vi "SetWindowIcon.vi"(7 "Action":enum16{"Set", "Reset"}(ring), 8 "error in (no error)":errorcluster, 10 "VIRef (calling VI)":refnum<vi>, 11 "ICO Icon":path) -> (0 "Error Out":errorcluster)   [LabVIEW 2022 SP3]
doc: "Set a custom title bar icon for the referenced VI.\nIf no VI reference is supplied the VI calling this function is altered.\n\nUse <b>set</b> to change the icon to a custom icon, and <b>reset</b> to revert the icon to the previous value."
uses:
  user32.dll
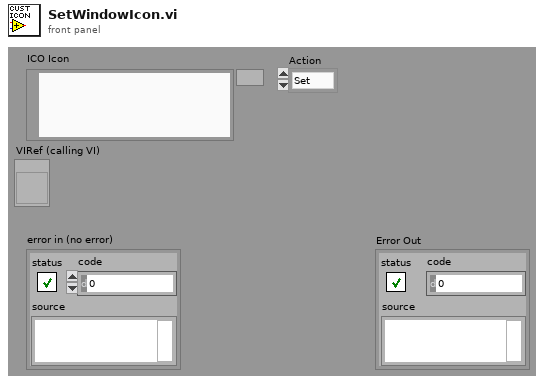
[diagram p1: front panel]
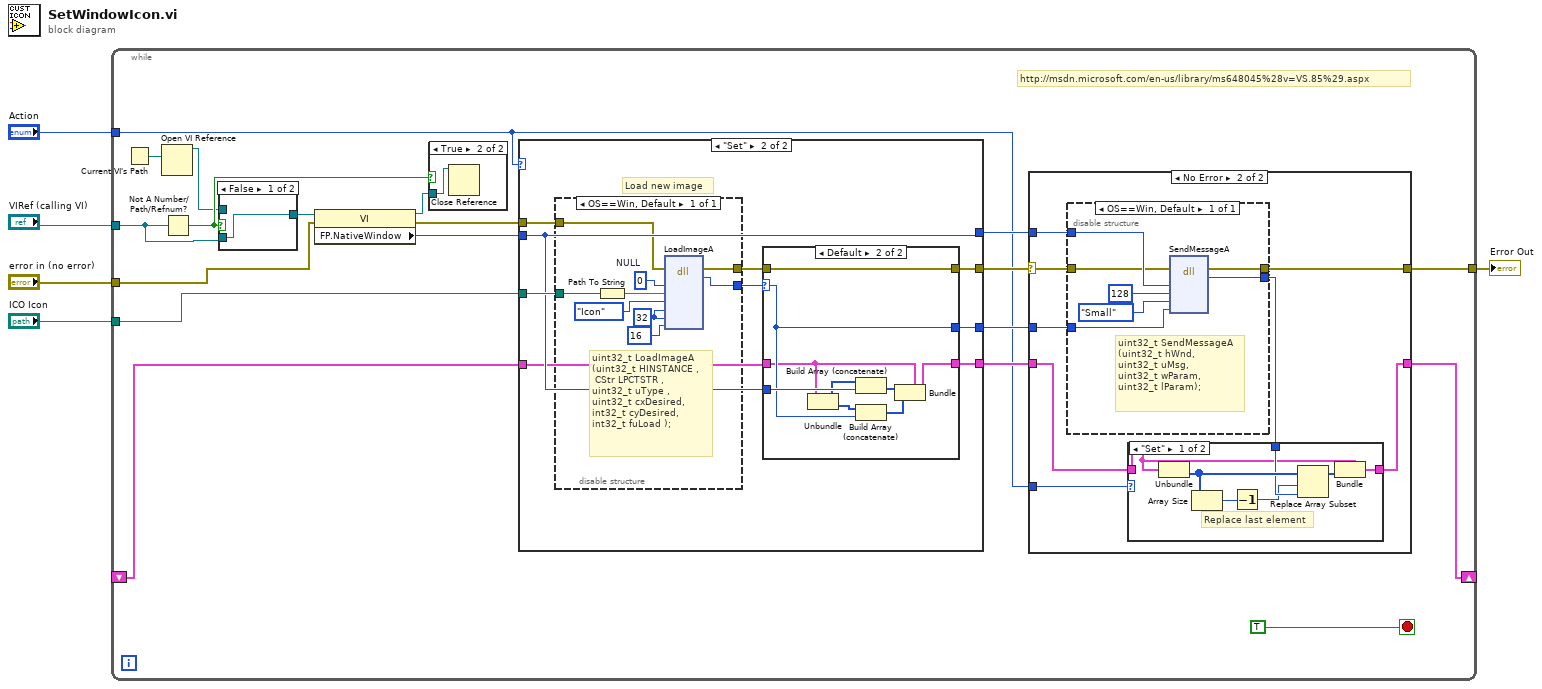
[diagram p0: block diagram]
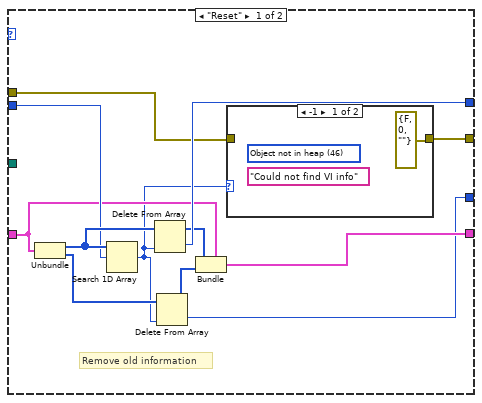
[diagram p3: hidden frame]
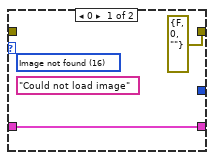
[diagram p5: hidden frame]
diagram:
  n1 = while {
    tunnel: "ICO Icon" -> [w24]
    tunnel: "error in (no error)" -> [w22]
    tunnel: "VIRef (calling VI)" -> [w7]
    tunnel: "Action" -> [w12]
    tunnel: [w16] -> w1
    shift-right: [w10] -> _
    shift-left: _ -> [w11]
    stop <- TRUE stop-if-true
    # "http://msdn.microsoft.com/en-us/library/ms648045%28v=VS.85%29.aspx"
    n2 = Current VI's Path() -> (path=w9:path)
    n3 = Open VI Reference(vi path=w9) -> (vi reference=w6:refnum<vi>)  [unwired: 5 in, 1 out]
    n4 = Not A Number/Path/Refnum?(number/path/refnum=w7) -> (NaN/Path/Refnum?=w14:bool)
    n5 = case shown="False" w14 {
      tunnel: [w69 w70] -> w8
      tunnel: w6 -> [_ w70]
      tunnel: w7 -> [w69 _]
      frame False {
      }
      frame True {
      }
    }
    n6 = property on="Property Node" class="VI"(reference=w8, error in=w22) -> (reference out=w15:refnum<vi>, error out=w21:errorcluster, "FP.NativeWindow"=w20:u64)
    n7 = case shown="True" w14 {
      tunnel: w15 -> [_ w25]
      frame False {
      }
      frame True {
        n8 = Close Reference(reference=w25) -> ()  [unwired: 1 in, 1 out]
      }
    }
    n9 = case shown="\"Set\"" w12 {
      tunnel: w24 -> [_ w48]
      tunnel: [w26 w44] -> w18
      tunnel: [w29 w45] -> w17
      tunnel: w21 -> [w27 w47]
      tunnel: [w35 w42] -> w19
      tunnel: w20 -> [w36 w42]
      tunnel: w11 -> [w31 w41]
      tunnel: [w30 w40] -> w13
      frame "Reset" {
        # "Remove old information"
        n10 = Unbundle(w31) -> (w37:u64[], w34:u32[])
        n11 = Search 1D Array(1D array=w37, element=w36) -> (index of element=w28:i32)  [unwired: 1 in]
        n12 = Delete From Array(array=w37, index=w28) -> (deleted portion=w35:u64, array with subset deleted=w33:u64[])  [unwired: 1 in]
        n13 = Delete From Array(array=w34, index=w28) -> (deleted portion=w29:u32, array with subset deleted=w32:u32[])  [unwired: 1 in]
        n14 = Bundle(cluster=w31, w33, w32) -> (w30:cluster{u64[], u32[]})
        n15 = case shown="-1" w28 {
          tunnel: [errorcluster {"status"=FALSE, "code"=0, "source"=""} ("error out") w39] -> w26
          tunnel: w27 -> [_ w39]
          frame -1 {
            (unwired) "Could not find VI info" ("source")
            (unwired) 46 items=["No error", "Argument error", "Memory is full", "Out of zone", "End of file", "File already open", "Generic file I/O error", "File not found", "File permission error", "Disk is full", "Duplicate path", "Too many files open", "System feature not enabled", "Resource file not found", "Cannot add resource", "Resource not found", "Image not found", "Image memory error", "Pen does not exist", "Config type invalid", "Config token not found", "Config parse error", "Config memory error", "Bad external code format", "Bad external code offset", "External code not present", "Null window", "Destroy window error", "Null menu", "Print aborted", "Bad print record", "Print driver error", "Windows error during printing", "Memory error during printing", "Print dialog error", "Generic print error", "Invalid device refnum", "Device not found", "Device parameter error", "Device unit error", "Cannot open device", "Device call aborted", "Generic error", "Cancelled by user", "Object ID too low", "Object ID too high", "Object not in heap", "Unknown heap", "Unknown object (invalid DefProc)", "Unknown object (DefProc not in table)", "Message out of range", "Invalid (null) method", "Unknown message", "Manager call not supported", "Bad address", "Network operation in progress", "Network operation timed out", "Connection is busy", "Network attribute not supported", "Network error", "Address in use", "System out of memory", "Connection aborted", "Connection refused", "Not connected", "Already connected", "Connection closed", "Initialization error (interapplication manager)", "Bad occurrence", "Wait on unbound occurrence handler", "Occurrence queue overflow", "Datalog type conflict", "Unused", "Unrecognized type (interapplication manager)", "Memory corrupt", "Failed to make temporary DLL", "Old CIN version", "Drag socket not found", "Failed to load drop-object", "Failed to register OLE object", "Failed to release OLE object", "Format specifier type mismatch", "Unknown format specifier", "Too few format specifiers", "Too many format specifiers", "Scan failed", "Newer CIN version", "Error converting to variant", "Runtime menu error", "Password tampered", "Variant attribute not found", "Incompatible variant data type", "Event data is not available", "Event Store is not present", "Occurrence is not found", "Event Queue is not created", "Event info is not available", "Refnum passed is NULL", "Error retrieving Class GUID", "Error retrieving CoClass GUID", "Error retrieving TypeLib GUID.", "Bad built application magic bytes.", "Specific driver is different from the specific driver associated with the Logical Name.", "There is no session opened to the class driver.", "Max Error", "MAX - Error with config objects", "MAX - Error loading configuration", "MAX - Group not supported"]
          }
          frame Default {
          }
        }
      }
      frame "Set" {
        # "Load new image"
        n16 = disable-structure "Conditional Disable Structure" shown="OS==Win, Default" {
          disable-tunnel: w48 -> [w54]
          disable-tunnel: w47 -> [w50]
          disable-tunnel: [w51] -> w46
          disable-tunnel: [w49] -> w43
          frame condition #0 (active) {
            w56 = u32 32 ("cxDesired")
            w57 = u32 0  # NULL
            # "uint32_t LoadImageA\n(uint32_t HINSTANCE ,\n CStr LPCTSTR ,\nuint32_t uType , \nuint32_t cxDesired, \nint32_t cyDesired, \nint32_t fuLoad );"
            n17 = Path To String(path=w54) -> (string=w53:string)
            n18 = dll-call lib="user32.dll" fn="LoadImageA" label="LoadImage"(error in=w50, "HINSTANCE"=w57, "LPCTSTR"=w53, "uType"=enum16{"Bitmap", "Icon", "Cursor"}."Icon", "cxDesired"=w56, "cyDesired"=w56, "fuLoad"=16) -> (error out=w49:errorcluster, "ImageHandle"=w51:u32)  [unwired: 8 in, 1 out]
          }
        }
        n19 = case shown="Default" w46 {
          selector: w46 -> [_ w66]
          tunnel: [_ w66] -> w45
          tunnel: [errorcluster {"status"=FALSE, "code"=0, "source"=""} ("error out") w68] -> w44
          tunnel: w43 -> [_ w68]
          tunnel: w42 -> [_ w67]
          tunnel: w41 -> [w59 w62]
          tunnel: [w59 w63] -> w40
          frame 0 {
            (unwired) "Could not load image" ("source")
            (unwired) 16 items=["No error", "Argument error", "Memory is full", "Out of zone", "End of file", "File already open", "Generic file I/O error", "File not found", "File permission error", "Disk is full", "Duplicate path", "Too many files open", "System feature not enabled", "Resource file not found", "Cannot add resource", "Resource not found", "Image not found", "Image memory error", "Pen does not exist", "Config type invalid", "Config token not found", "Config parse error", "Config memory error", "Bad external code format", "Bad external code offset", "External code not present", "Null window", "Destroy window error", "Null menu", "Print aborted", "Bad print record", "Print driver error", "Windows error during printing", "Memory error during printing", "Print dialog error", "Generic print error", "Invalid device refnum", "Device not found", "Device parameter error", "Device unit error", "Cannot open device", "Device call aborted", "Generic error", "Cancelled by user", "Object ID too low", "Object ID too high", "Object not in heap", "Unknown heap", "Unknown object (invalid DefProc)", "Unknown object (DefProc not in table)", "Message out of range", "Invalid (null) method", "Unknown message", "Manager call not supported", "Bad address", "Network operation in progress", "Network operation timed out", "Connection is busy", "Network attribute not supported", "Network error", "Address in use", "System out of memory", "Connection aborted", "Connection refused", "Not connected", "Already connected", "Connection closed", "Initialization error (interapplication manager)", "Bad occurrence", "Wait on unbound occurrence handler", "Occurrence queue overflow", "Datalog type conflict", "Unused", "Unrecognized type (interapplication manager)", "Memory corrupt", "Failed to make temporary DLL", "Old CIN version", "Drag socket not found", "Failed to load drop-object", "Failed to register OLE object", "Failed to release OLE object", "Format specifier type mismatch", "Unknown format specifier", "Too few format specifiers", "Too many format specifiers", "Scan failed", "Newer CIN version", "Error converting to variant", "Runtime menu error", "Password tampered", "Variant attribute not found", "Incompatible variant data type", "Event data is not available", "Event Store is not present", "Occurrence is not found", "Event Queue is not created", "Event info is not available", "Refnum passed is NULL", "Error retrieving Class GUID", "Error retrieving CoClass GUID", "Error retrieving TypeLib GUID.", "Bad built application magic bytes.", "Specific driver is different from the specific driver associated with the Logical Name.", "There is no session opened to the class driver.", "Max Error", "MAX - Error with config objects", "MAX - Error loading configuration", "MAX - Group not supported"]
          }
          frame Default {
            n20 = Unbundle(w62) -> (w61:u64[], w60:u32[])
            n21 = Build Array (concatenate)(w61, w67) -> (w65:u64[])
            n22 = Build Array (concatenate)(w60, w66) -> (w64:u32[])
            n23 = Bundle(cluster=w62, w65, w64) -> (w63:cluster{u64[], u32[]})
          }
        }
      }
    }
    n24 = case shown="No Error" w18 {
      selector: w18 -> [w72 w77]
      tunnel: [w72 w80] -> w16
      tunnel: w19 -> [_ w79]
      tunnel: w17 -> [_ w78]
      tunnel: w13 -> [w71 w74]
      tunnel: [w71 w75] -> w10
      tunnel: w12 -> [_ w73]
      frame Error {
      }
      frame No Error {
        n25 = disable-structure "Conditional Disable Structure" shown="OS==Win, Default" {
          disable-tunnel: [w89] -> w80
          disable-tunnel: w79 -> [w94]
          disable-tunnel: w78 -> [w92]
          disable-tunnel: w77 -> [w90]
          disable-tunnel: [w91] -> w76
          frame condition #0 (active) {
            # "uint32_t SendMessageA\n(uint32_t hWnd,\nuint32_t uMsg,\nuint32_t wParam,\nuint32_t lParam);"
            n26 = dll-call lib="user32.dll" fn="SendMessageA" label="SendMessage"(error in=w90, "hWnd"=w94, "uMsg"=128 ("dimension size"), "wParam"=enum16{"Small", "Big"}."Small", "lParam"=w92) -> (error out=w89:errorcluster, "OldHandle"=w91:u32)  [unwired: 6 in, 1 out]
          }
        }
        n27 = case shown="\"Set\"" w73 {
          tunnel: w76 -> [w86 _]
          tunnel: [w82 w88] -> w75
          tunnel: w74 -> [w81 w88]
          frame "Set" {
            # "Replace last element"
            n28 = Unbundle(w81) -> (w87:u32[])  [unwired: 1 out]
            n29 = Array Size(array=w87) -> (size(s)=w85:i32)
            n30 = Decrement(x=w85) -> (x-1=w84:i32)
            n31 = Replace Array Subset(array=w87, new element=w86, index=w84) -> (w83:u32[])
            n32 = Bundle(cluster=w81, w83) -> (w82:cluster{u64[], u32[]})  [unwired: 1 in]
          }
          frame "Reset" {
          }
        }
      }
    }
  }
  "Error Out" <- w1
